vi "p2.vi"() -> ()   [LabVIEW 2023, in "d3.lvlib"]
uses:
  d3.lvlib
  38863839-b270-4a4a-9785-24c709bd974d.vi
  AOC/AOC.lvlib
panel:
  in  "Example":string="467..114..\n...*......\n..35..633.\n......#...\n617*......\n.....+.58.\n..592.....\n......755.\n...$.*....\n.664.598.."
  in  "Example":bool
  out "Answer":i64=7746
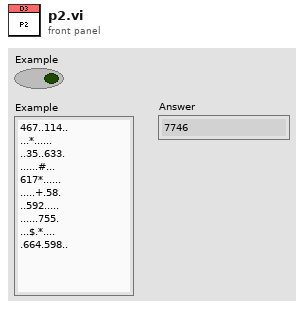
[diagram p1: front panel]
types:
  T1 = cluster{i64, "array with duplicates removed":cluster{i32, i32}[]}
  T2 = cluster{i64, "array with duplicates removed":cluster{i32, i32}[]}[]
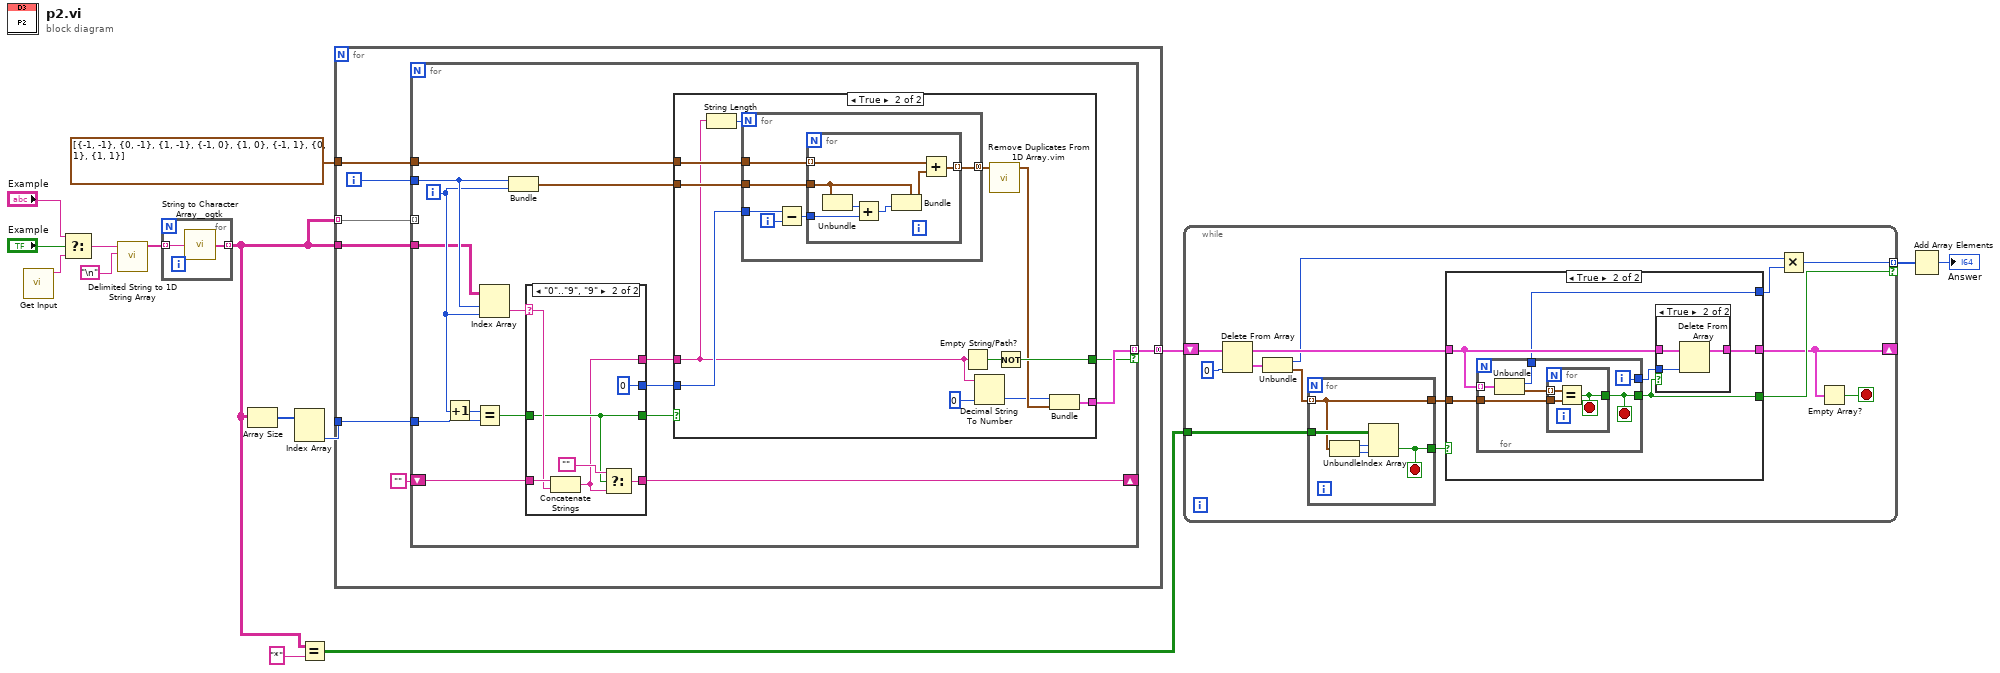
[diagram p0: block diagram]
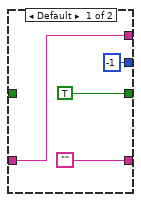
[diagram p5: hidden frame]
diagram:
  n1 = call "Get Input.vi"() -> ("Input"=w14:string)  [unwired: 11 in]
  n2 = Select(t="Example", s="Example", f=w14) -> (s? t:f=w11:string)
  n3 = call <vilib>:"Delimited String to 1D String Array.vi"("delimiter"="\n", "delimited string"=w11) -> ("string array"=w10:string[])  [unwired: 9 in]
  n4 = for {
    tunnel: w10 -> [w17] mode=indexing
    tunnel: [w16] -> w4 mode=indexing
    n5 = call <userlib>:"String to Character Array__ogtk.vi"("Input String"=w17) -> ("Character Array"=w16:string[])
  }
  n6 = Array Size(array=w4) -> (size(s)=w8:i32[])
  n7 = Index Array(array=w8) -> (element #2=w7:i32)  [unwired: 2 in, 1 out]
  n8 = Equal?(x=w4, y="*") -> (x = y?=w2:bool[][])
  n9 = for {
    tunnel: w4 -> [w21]
    tunnel: w7 -> [w23]
    tunnel: cluster{i32, i32}[] [{-1, -1}, {0, -1}, {1, -1}, {-1, 0}, {1, 0}, {-1, 1}, {0, 1}, {1, 1}] -> [w22]
    tunnel: w4 -> [w19] mode=indexing
    tunnel: [w18] -> w5 mode=concatenating
    i -> [w20]
    n10 = for {
      tunnel: w21 -> [w32]
      tunnel: w20 -> [w35]
      shift-right: [w28] -> _
      shift-left: "" ("String") -> [w40]
      tunnel: w23 -> [w37]
      tunnel: w22 -> [w36]
      tunnel: [w27] -> w18 mode=indexing if=w25
      tunnel: w19 -> [_] mode=indexing
      i -> [w34]
      n11 = Increment(x=w34) -> (x+1=w38:i32)
      n12 = Equal?(x=w38, y=w37) -> (x = y?=w26:bool)
      n13 = Index Array(array=w32, index (row)=w35, index (col)=w34) -> (element=w39:string)
      n14 = Bundle(w35, w34) -> (w33:cluster{i32, i32})  [unwired: 1 in]
      n15 = case shown="\"0\"..\"9\", \"9\"" w39 {
        selector: w39 -> [_ w75]
        tunnel: w40 -> [w68 w76]
        tunnel: ["" w74] -> w28
        tunnel: w26 -> [_ w72]
        tunnel: [TRUE w72] -> w29
        tunnel: [w68 w71] -> w31
        tunnel: [-1 0] -> w30
        frame Default {
        }
        frame "0".."9", "9" {
          n16 = Concatenate Strings(w76, w75) -> (w71:string)
          n17 = Select(t="", s=w72, f=w71) -> (s? t:f=w74:string)
        }
      }
      n18 = case shown="True" w29 {
        tunnel: w36 -> [_ w52]
        tunnel: w33 -> [_ w51]
        tunnel: w31 -> [_ w45]
        tunnel: w30 -> [_ w50]
        tunnel: [_ w41] -> w27
        tunnel: [_ w47] -> w25
        frame False {
        }
        frame True {
          n19 = String Length(string=w45) -> (length=w49:i32)
          n20 = for {
            N: w49 -> [_]
            tunnel: w52 -> [w58]
            tunnel: w51 -> [w57]
            tunnel: w50 -> [w56]
            tunnel: [w53] -> w44 mode=concatenating
            i -> [w54]
            n21 = Subtract(x=w56, y=w54) -> (x-y=w55:i32)
            n22 = for {
              tunnel: w58 -> [w65] mode=indexing
              tunnel: w57 -> [w63]
              tunnel: w55 -> [w61]
              tunnel: [w59] -> w53 mode=indexing
              n23 = Unbundle(w63) -> (w62:i32)  [unwired: 1 out]
              n24 = Add(x=w62, y=w61) -> (x+y=w60:i32)
              n25 = Bundle(cluster=w63, w60) -> (w64:cluster{i32, i32})  [unwired: 1 in]
              n26 = Add(x=w65, y=w64) -> (x+y=w59:cluster{i32, i32})
            }
          }
          n27 = Empty String/Path?(string/path=w45) -> (empty?=w48:bool)
          n28 = Decimal String To Number(string=w45, default (0L)=i64 0 ("Answer")) -> (number=w42:i64)  [unwired: 1 in, 1 out]
          n29 = call "Remove Duplicates From 1D Array.vim"("array"=w44) -> ("array with duplicates removed"=w43:cluster{i32, i32}[])  [unwired: 10 in]
          n30 = Not(x=w48) -> (.not. x?=w47:bool)
          n31 = Bundle(w42, "array with duplicates removed"=w43) -> (w41:T1)  [unwired: 1 in]
        }
      }
    }
  }
  n32 = while {
    tunnel: w2 -> [w87]
    shift-right: [w78] -> _
    shift-left: w5 -> [w90]
    tunnel: [w80] -> w1 mode=indexing if=w79
    stop <- w77 stop-if-true
    n33 = Delete From Array(array=w90, index=0) -> (deleted portion=w88:T1, array with subset deleted=w85:T2)  [unwired: 1 in]
    n34 = Unbundle(w88) -> (w81:i64, "array with duplicates removed"=w84:cluster{i32, i32}[])
    n35 = for {
      tunnel: w84 -> [w111] mode=indexing
      tunnel: w87 -> [w115]
      tunnel: [w112] -> w86
      tunnel: [w111] -> w83
      stop <- w112 stop-if-true
      n36 = Unbundle(w111) -> (w114:i32, w113:i32)
      n37 = Index Array(array=w115, index (row)=w114, index (col)=w113) -> (element=w112:bool)
    }
    n38 = case shown="True" w86 {
      tunnel: w85 -> [w91 w96]
      tunnel: w83 -> [_ w97]
      tunnel: [w91 w94] -> w78
      tunnel: [_ w93] -> w82
      tunnel: [_ w92] -> w79
      frame False {
      }
      frame True {
        n39 = for {
          tunnel: w96 -> [w107] mode=indexing
          tunnel: w97 -> [w105]
          tunnel: [w104] -> w95
          tunnel: [w103] -> w92
          tunnel: [w102] -> w93
          i -> [w104]
          stop <- w103 stop-if-true
          n40 = Unbundle(w107) -> (w102:i64, "array with duplicates removed"=w106:cluster{i32, i32}[])
          n41 = for {
            tunnel: w106 -> [w110] mode=indexing
            tunnel: w105 -> [w109]
            tunnel: [w108] -> w103
            stop <- w108 stop-if-true
            n42 = Equal?(x=w110, y=w109) -> (x = y?=w108:bool)
          }
        }
        n43 = case shown="True" w92 {
          tunnel: w96 -> [w98 w101]
          tunnel: w95 -> [_ w100]
          tunnel: [w98 w99] -> w94
          frame False {
          }
          frame True {
            n44 = Delete From Array(array=w101, index=w100) -> (array with subset deleted=w99:T2)  [unwired: 1 in, 1 out]
          }
        }
      }
    }
    n45 = Multiply(x=w81, y=w82) -> (x*y=w80:i64)
    n46 = Empty Array?(array=w78) -> (empty?=w77:bool)
  }
  n47 = Add Array Elements(numeric array=w1) -> (sum=→"Answer":i64)
